vi "lectura giroscopio.vi"(4 "read buffer":string) -> (0 "Giroscopio Z":i32[](array[numeric]), 1 "Giroscopio Y":i32[](array[numeric]), 2 "Giroscopio X":i32[](array[numeric]))   [LabVIEW 2020]
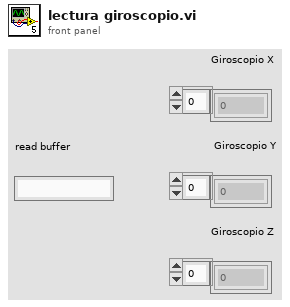
[diagram p1: front panel]
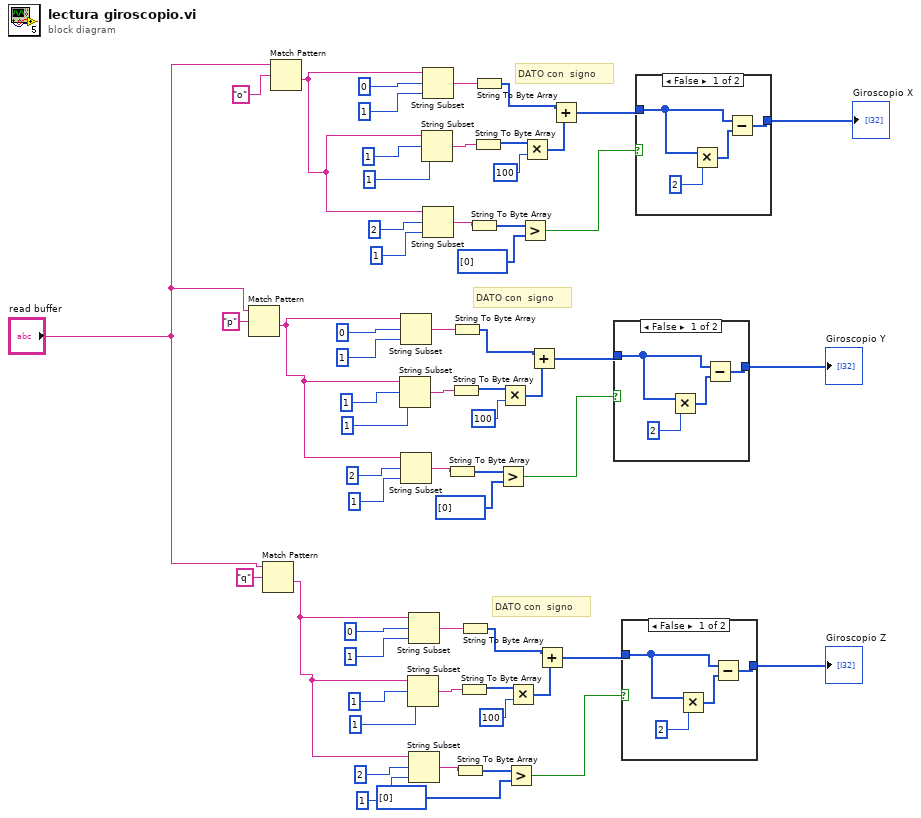
[diagram p0: block diagram]
diagram:
  # "DATO con  signo"
  # "DATO con  signo"
  # "DATO con  signo"
  n1 = Match Pattern(string="read buffer", regular expression="p") -> (after substring=w39:string)  [unwired: 1 in, 3 out]
  n2 = Match Pattern(string="read buffer", regular expression="q") -> (after substring=w58:string)  [unwired: 1 in, 3 out]
  n3 = Match Pattern(string="read buffer", regular expression="o") -> (after substring=w20:string)  [unwired: 1 in, 3 out]
  n4 = String Subset(string=w39, offset (0)=1, length (rest)=1 ("length (rest)")) -> (substring=w29:string)
  n5 = String Subset(string=w39, offset (0)=0, length (rest)=1 ("length (rest)")) -> (substring=w30:string)
  n6 = String Subset(string=w39, offset (0)=2, length (rest)=1 ("length (rest)")) -> (substring=w24:string)
  n7 = String Subset(string=w58, offset (0)=1, length (rest)=1 ("length (rest)")) -> (substring=w48:string)
  n8 = String Subset(string=w58, offset (0)=0, length (rest)=1 ("length (rest)")) -> (substring=w49:string)
  n9 = String Subset(string=w58, offset (0)=2, length (rest)=1 ("length (rest)")) -> (substring=w43:string)
  n10 = String Subset(string=w20, offset (0)=1, length (rest)=1 ("length (rest)")) -> (substring=w10:string)
  n11 = String Subset(string=w20, offset (0)=0, length (rest)=1 ("length (rest)")) -> (substring=w11:string)
  n12 = String Subset(string=w20, offset (0)=2, length (rest)=1 ("length (rest)")) -> (substring=w5:string)
  n13 = String To Byte Array(string=w24) -> (unsigned byte array=w23:u8[])
  n14 = String To Byte Array(string=w29) -> (unsigned byte array=w28:u8[])
  n15 = String To Byte Array(string=w30) -> (unsigned byte array=w25:u8[])
  n16 = String To Byte Array(string=w43) -> (unsigned byte array=w42:u8[])
  n17 = String To Byte Array(string=w48) -> (unsigned byte array=w47:u8[])
  n18 = String To Byte Array(string=w49) -> (unsigned byte array=w44:u8[])
  n19 = String To Byte Array(string=w5) -> (unsigned byte array=w4:u8[])
  n20 = String To Byte Array(string=w10) -> (unsigned byte array=w9:u8[])
  n21 = String To Byte Array(string=w11) -> (unsigned byte array=w6:u8[])
  n22 = Greater?(x=w23, y=u8[] [0]) -> (0:w21:bool)
  n23 = Multiply(x=w28, y=100) -> (x*y=w26:i32[])
  n24 = Greater?(x=w42, y=u8[] [0]) -> (0:w40:bool)
  n25 = Multiply(x=w47, y=100) -> (x*y=w45:i32[])
  n26 = Greater?(x=w4, y=u8[] [0]) -> (0:w2:bool)
  n27 = Multiply(x=w9, y=100) -> (x*y=w7:i32[])
  n28 = Add(x=w25, y=w26) -> (x+y=w37:i32[])
  n29 = Add(x=w44, y=w45) -> (x+y=w56:i32[])
  n30 = Add(x=w6, y=w7) -> (x+y=w18:i32[])
  n31 = case shown="False" w21 {
    tunnel: w37 -> [w64 w66]
    tunnel: [w63 w66] -> w60
    frame False {
      n32 = Multiply(x=w64, y=2) -> (x*y=w65:i32[])
      n33 = Subtract(x=w64, y=w65) -> (x-y=w63:i32[])
    }
    frame True {
    }
  }
  "Giroscopio Y" <- w60
  n34 = case shown="False" w40 {
    tunnel: w56 -> [w69 w71]
    tunnel: [w68 w71] -> w61
    frame False {
      n35 = Multiply(x=w69, y=2) -> (x*y=w70:i32[])
      n36 = Subtract(x=w69, y=w70) -> (x-y=w68:i32[])
    }
    frame True {
    }
  }
  "Giroscopio Z" <- w61
  n37 = case shown="False" w2 {
    tunnel: w18 -> [w74 w76]
    tunnel: [w73 w76] -> w59
    frame False {
      n38 = Multiply(x=w74, y=2) -> (x*y=w75:i32[])
      n39 = Subtract(x=w74, y=w75) -> (x-y=w73:i32[])
    }
    frame True {
    }
  }
  "Giroscopio X" <- w59
